vi "counter_rate.vi"(10 "channel":u64, 11 "file (use dialog)":path) -> (0 "error out":errorcluster, 1 "cal":u64[](graph), 2 "diff":u64[](array[numeric]), 3 "data":u64[](array[numeric]) format="%x")   [LabVIEW 2017]
panel:
  out "data 5":string
  out "channel number":u64 format="%x"
  out "number 3":u32
  out "substring":string
  out "number 2":u64 format="%x"
  out "x*y":dbl[](array[numeric])
  out "number":u64 format="%x"
  out "data 4":string
  out "data 3":string
  out "data 2":string
  out "data":string
  # "G:\\tdc\\2017\\test_20231106_044219.dat"
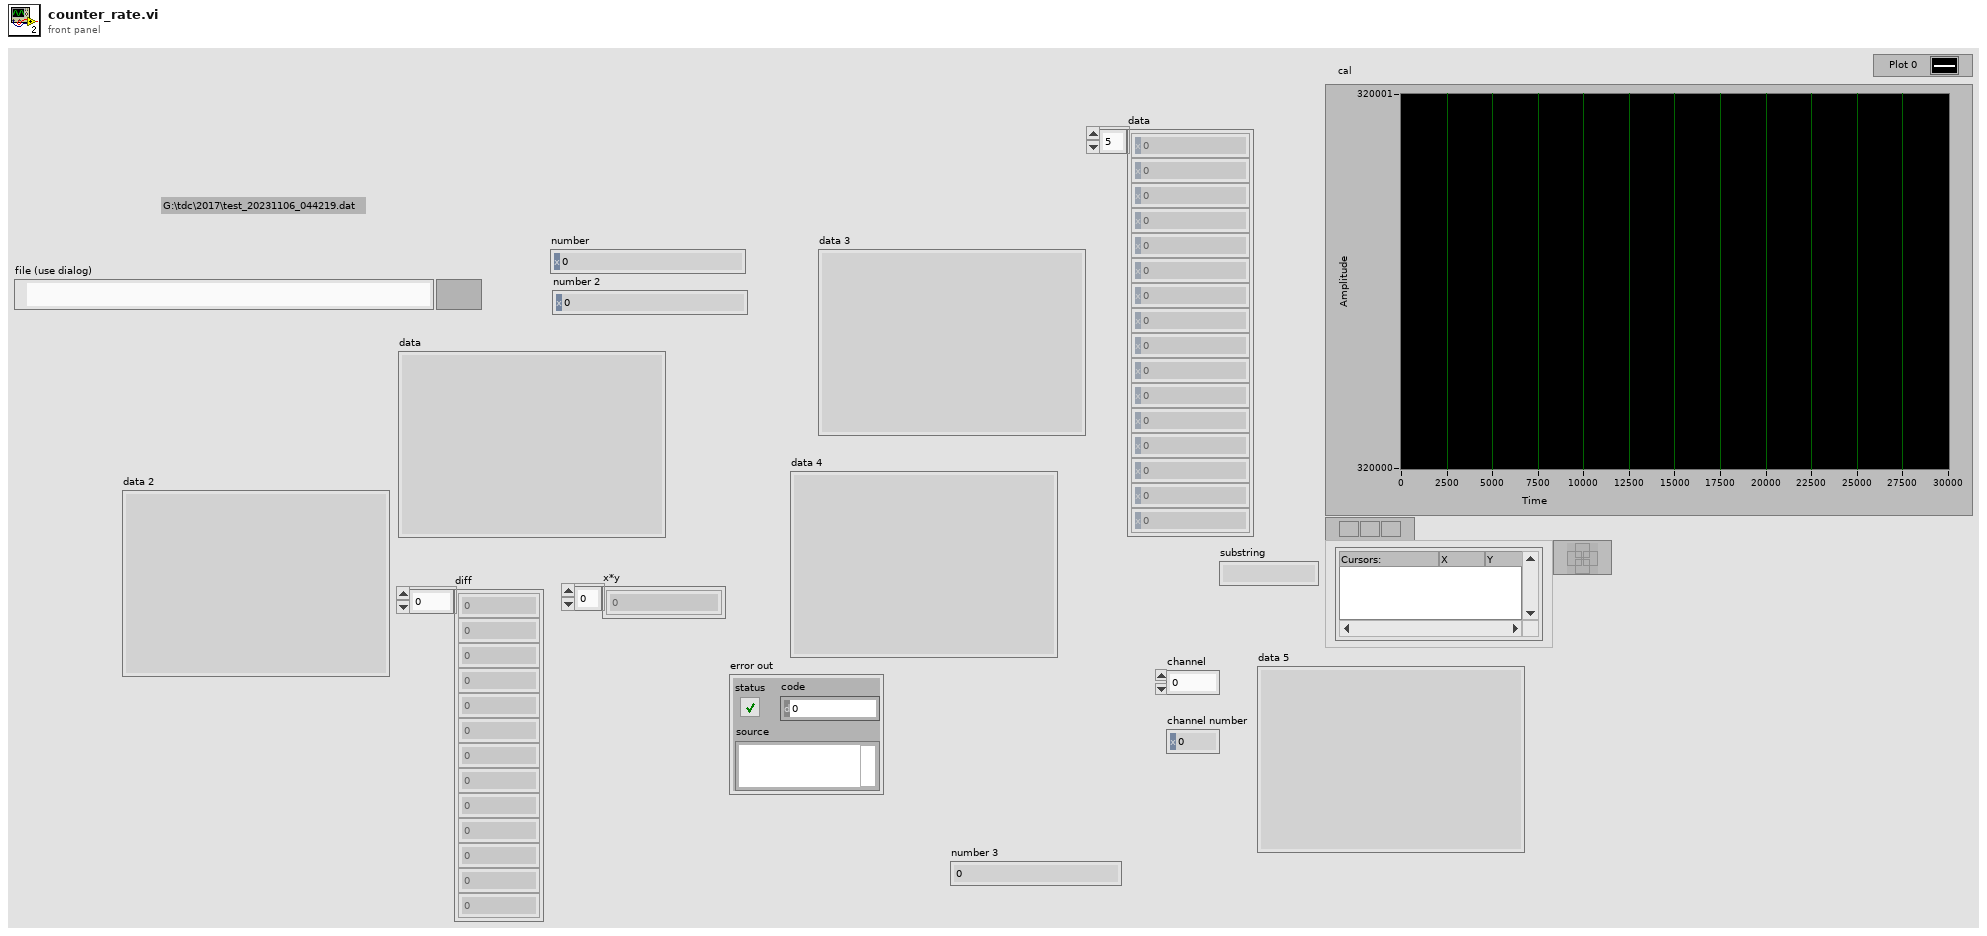
[diagram p1: front panel]
types:
  T1 = enum16{"open", "replace", "create", "open or create", "replace or create", "replace or create with confirmation"}
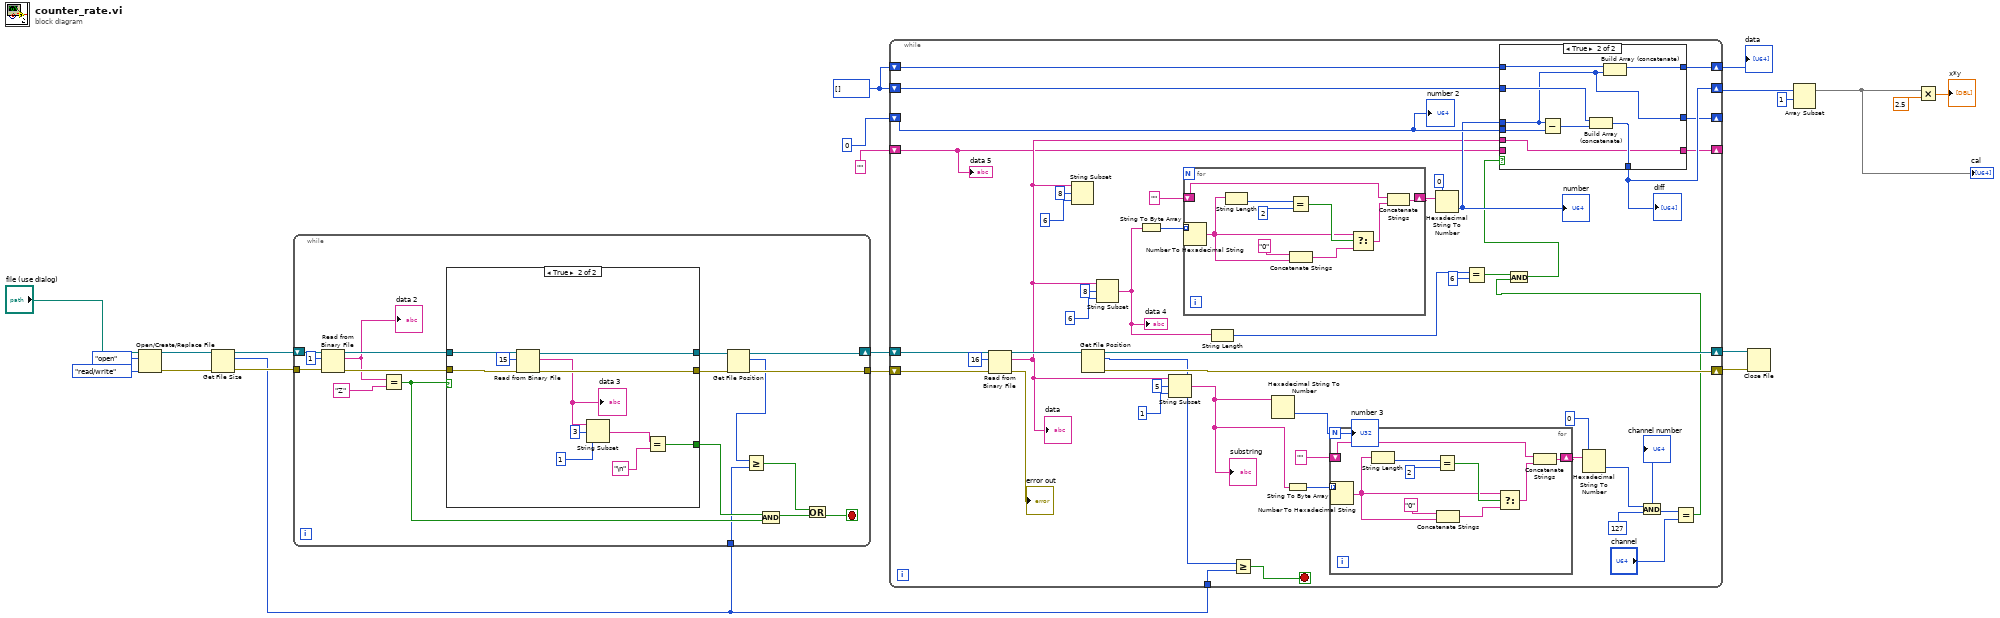
[diagram p0: block diagram]
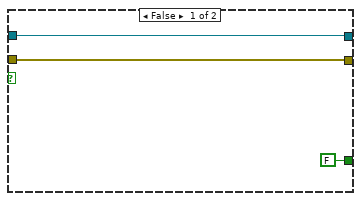
[diagram p3: hidden frame]
diagram:
  w5 = u64[] []
  n1 = Open/Create/Replace File(file path (use dialog)="file (use dialog)", operation (0:open)=T1."open", access (0:read/write)=enum16{"read/write", "read-only", "write-only"}."read/write") -> (refnum out=w20:refnum<file>, error out=w14:errorcluster)  [unwired: 3 in, 1 out]
  n2 = Get File Size(file=w20, error in=w14) -> (refnum out=w15:refnum<file>, size (in bytes)=w1:i64, 0:w13:errorcluster)
  n3 = while {
    tunnel: w13 -> [w38]
    shift-right: [w26] -> w16
    shift-left: w15 -> [w39]
    tunnel: [w27] -> w17
    tunnel: w1 -> [w25]
    stop <- w23 stop-if-true
    n4 = Read from Binary File(8:w38, 10:1 ("count (1)"), 11:w39) -> (0:w34:errorcluster, 2:w32:string, 3:w35:refnum<file>)  [unwired: 3 in, 1 out]
    "data 2" <- w32
    n5 = Equal?(x=w32, y="Z") -> (x = y?=w29:bool)
    n6 = case shown="True" w29 {
      tunnel: w35 -> [w42 w53]
      tunnel: w34 -> [w41 w52]
      tunnel: [w42 w50] -> w33
      tunnel: [w41 w49] -> w28
      tunnel: [FALSE w43] -> w30
      frame False {
      }
      frame True {
        n7 = Read from Binary File(8:w52, 10:15 ("count (1)"), 11:w53) -> (0:w49:errorcluster, 2:w46:string, 3:w50:refnum<file>)  [unwired: 3 in, 1 out]
        "data 3" <- w46
        n8 = String Subset(string=w46, offset (0)=3, length (rest)=1 ("length (rest)")) -> (substring=w45:string)
        n9 = Equal?(x=w45, y="\n") -> (x = y?=w43:bool)
      }
    }
    n10 = Get File Position(4:w28, 7:w33) -> (0:w27:errorcluster, 2:w24:i64, 3:w26:refnum<file>)
    n11 = Greater Or Equal?(x=w24, y=w25) -> (x >= y?=w22:bool)
    n12 = Compound Arithmetic op=AND(w30, w29) -> (w31:bool)
    n13 = Or(x=w22, y=w31) -> (x .or. y?=w23:bool)
  }
  n14 = while {
    shift-right: [w94] -> w12
    shift-left: w16 -> [w98]
    shift-right: [w96] -> w11
    shift-left: w17 -> [w99]
    tunnel: w1 -> [w92]
    shift-right: [w57] -> _
    shift-left: 0 ("length (rest)") -> [w71]
    shift-right: [w69] -> w10
    shift-left: w5 -> [w70]
    shift-right: [w58] -> w4
    shift-left: w5 -> [w59]
    shift-right: [w56] -> _
    shift-left: "" ("format string") -> [w54]
    stop <- w91 stop-if-true
    n15 = Read from Binary File(8:w99, 10:16 ("count (1)"), 11:w98) -> (0:→"error out":errorcluster, 2:w55:string, 3:w95:refnum<file>)  [unwired: 3 in, 1 out]
    "data" <- w55
    n16 = String Subset(string=w55, offset (0)=8, length (rest)=6 ("length (rest)")) -> ()  [unwired: 1 out]
    n17 = Get File Position(7:w95) -> (0:w96:errorcluster, 2:w93:i64, 3:w94:refnum<file>)  [unwired: 1 in]
    n18 = String Subset(string=w55, offset (0)=8, length (rest)=6 ("length (rest)")) -> (substring=w65:string)
    "data 4" <- w65
    n19 = String To Byte Array(string=w65) -> (unsigned byte array=w87:u8[])
    n20 = String Subset(string=w55, offset (0)=5, length (rest)=1 ("length (rest)")) -> (substring=w74:string)
    "substring" <- w74
    n21 = for {
      shift-right: [w130] -> w86
      shift-left: "" ("format string") -> [w127]
      tunnel: w87 -> [w131] mode=indexing
      n22 = Number To Hexadecimal String(2:w131) -> (0:w123:string)  [unwired: 1 in]
      n23 = String Length(string=w123) -> (length=w129:i32)
      n24 = Equal?(x=w129, y=2) -> (x = y?=w126:bool)
      n25 = Concatenate Strings("0" ("format string"), w123) -> (w125:string)
      n26 = Select(t=w123, s=w126, f=w125) -> (s? t:f=w122:string)
      n27 = Concatenate Strings(w127, w122) -> (w130:string)
    }
    n28 = String Length(string=w65) -> (length=w62:i32)
    n29 = Greater Or Equal?(x=w93, y=w92) -> (x >= y?=w91:bool)
    n30 = Hexadecimal String To Number(string=w74) -> (number=→"number 3":u32)  [unwired: 2 in, 1 out]
    n31 = String To Byte Array(string=w74) -> (unsigned byte array=w77:u8[])
    n32 = for {
      shift-right: [w120] -> w76
      shift-left: "" ("format string") -> [w117]
      tunnel: w77 -> [w121] mode=indexing
      n33 = Number To Hexadecimal String(2:w121) -> (0:w113:string)  [unwired: 1 in]
      n34 = String Length(string=w113) -> (length=w119:i32)
      n35 = Equal?(x=w119, y=2) -> (x = y?=w116:bool)
      n36 = Concatenate Strings("0" ("format string"), w113) -> (w115:string)
      n37 = Select(t=w113, s=w116, f=w115) -> (s? t:f=w112:string)
      n38 = Concatenate Strings(w117, w112) -> (w120:string)
    }
    n39 = Hexadecimal String To Number(string=w86, default (0uL)=u64 0 ("default (0 U32)")) -> (number=w68:u64)  [unwired: 1 in, 1 out]
    "number" <- w68
    n40 = Equal?(x=w62, y=6) -> (x = y?=w64:bool)
    n41 = Hexadecimal String To Number(string=w76, default (0uL)=u64 0 ("default (0 U32)")) -> (number=w73:u64)  [unwired: 1 in, 1 out]
    n42 = And(x=w73, y=u64 127 ("default (0 U32)")) -> (x .and. y?=w67:u64)
    "channel number" <- w67
    n43 = Equal?(x=w67, y="channel") -> (x = y?=w63:bool)
    n44 = And(x=w64, y=w63) -> (x .and. y?=w60:bool)
    n45 = case shown="True" w60 {
      tunnel: w71 -> [w101 w110]
      tunnel: w70 -> [w103 w109]
      tunnel: [w103 w108] -> w69
      tunnel: w68 -> [_ w105]
      tunnel: w59 -> [w102 w107]
      tunnel: [w102 w106] -> w58
      tunnel: [w101 w105] -> w57
      tunnel: w54 -> [w100 _]
      tunnel: [w100 w104] -> w56
      tunnel: w55 -> [_ w104]
      frame False {
      }
      frame True {
        n46 = Subtract(x=w105, y=w110) -> (x-y=w111:u64)
        n47 = Build Array (concatenate)(w109, w111) -> (w108:u64[])
        n48 = Build Array (concatenate)(w107, w105) -> (w106:u64[])
      }
    }
    "diff" <- w69
    "number 2" <- w71
    "data 5" <- w54
  }
  "data" <- w4
  n49 = Close File(refnum=w12, error in=w11) -> ()  [unwired: 2 out]
  n50 = Array Subset(array=w10, index=1) -> (w3:u64[])  [unwired: 1 in]
  "cal" <- w3
  n51 = Multiply(x=w3, y=2.5) -> (x*y=→"x*y":dbl[])
